vi "read current.vi"(8 "error in (no error)":errorcluster, 11 "PSP-603 in":refnum<class "PSP-603.lvclass">) -> (0 "error out":errorcluster, 2 "Current [A]":dbl, 3 "PSP-603 out":refnum<class "PSP-603.lvclass">)   [LabVIEW 2025, in "Power Supply.lvlib" / "PSP-603.lvclass"]
uses:
  PSP-603.lvclass
  PSP-603.lvclass/PSP-603.ctl
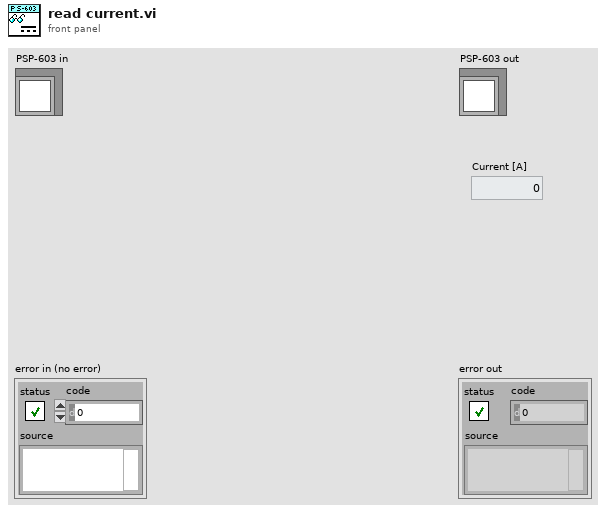
[diagram p1: front panel]
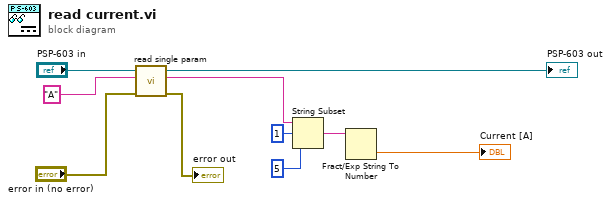
[diagram p0: block diagram]
diagram:
  n1 = call-dynamic "read single param.vi"("error in (no error)"="error in (no error)", "Parameter"="A", "PSP-603 in"="PSP-603 in") -> ("error out"=→"error out":errorcluster, "Data"=w2:string, "PSP-603 out"=→"PSP-603 out":refnum<class "PSP-603.lvclass">)  [unwired: 6 in]
  n2 = String Subset(string=w2, offset (0)=1, length (rest)=5 ("length (rest)")) -> (substring=w4:string)
  n3 = Fract/Exp String To Number(string=w4) -> (number=→"Current [A]":dbl)  [unwired: 3 in, 1 out]
